vi "TPD数据判定.vi"(7 "data in":u8[](array[numeric])) -> (8 "result":bool)   [LabVIEW 2016]
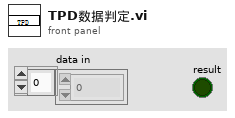
[diagram p1: front panel]
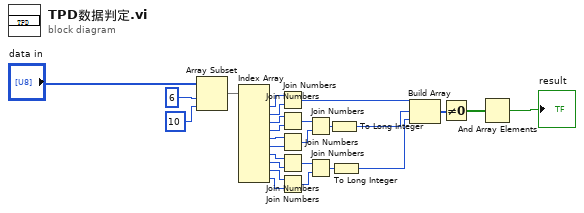
[diagram p0: block diagram]
diagram:
  n1 = Array Subset(array="data in", index=6, length=10) -> (w9:u8[])
  n2 = Index Array(array=w9) -> (element #1=w10:u8, element #2=w11:u8, element #3=w12:u8, element #4=w13:u8, element #5=w14:u8, element #6=w15:u8, element #7=w19:u8, element #8=w20:u8, element #9=w21:u8, element #10=w5:u8)  [unwired: 10 in]
  n3 = Join Numbers(hi=w10, lo=w11) -> ((hi.lo)=w24:u16)
  n4 = Join Numbers(hi=w12, lo=w13) -> ((hi.lo)=w16:u16)
  n5 = Join Numbers(hi=w14, lo=w15) -> ((hi.lo)=w17:u16)
  n6 = Join Numbers(hi=w19, lo=w20) -> ((hi.lo)=w18:u16)
  n7 = Join Numbers(hi=w21, lo=w5) -> ((hi.lo)=w4:u16)
  n8 = Join Numbers(hi=w16, lo=w17) -> ((hi.lo)=w22:u32)
  n9 = Join Numbers(hi=w18, lo=w4) -> ((hi.lo)=w23:u32)
  n10 = To Long Integer(number=w22) -> (32bit integer=w25:i32)
  n11 = To Long Integer(number=w23) -> (32bit integer=w26:i32)
  n12 = Build Array(w24, w25, w26) -> (w3:i32[])
  n13 = Not Equal To 0?(x=w3) -> (x != 0?=w2:bool[])
  n14 = And Array Elements(Boolean array=w2) -> (logical AND=→"result":bool)
